vi "Get User Interface VI.vi"(8 "error in (no error)":errorcluster, 11 "DSF Buffer Converter Transfers UI in":refnum<class "Default Buffer Converter Transfers UI.lvclass">) -> (0 "error out":errorcluster, 2 "user interface vi":refnum<vi>, 3 "DSF Buffer Converter Transfers UI out":refnum<class "Default Buffer Converter Transfers UI.lvclass">)   [LabVIEW 2020, in "DSF Core.lvlib" / "Default Buffer Converter Transfers UI.lvclass"]
uses:
  Default Buffer Converter Transfers UI.lvclass
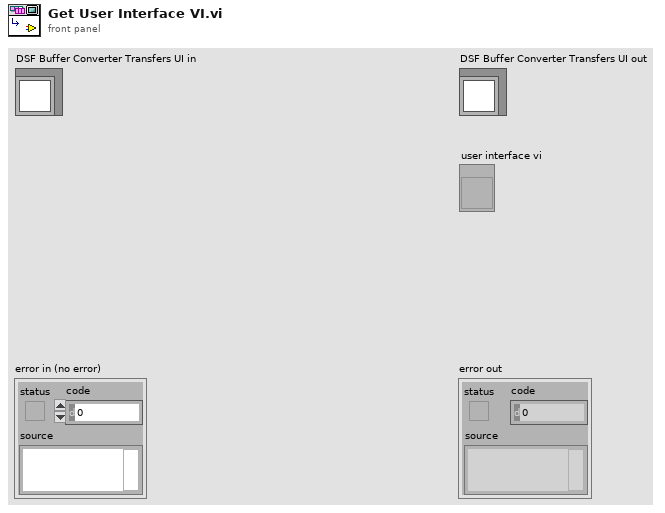
[diagram p1: front panel]
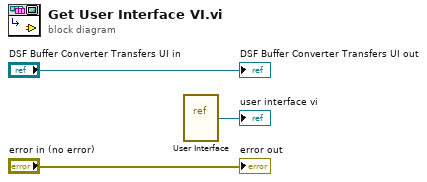
[diagram p0: block diagram]
diagram:
  n1 = vi-ref "User Interface.vi"() -> (→"user interface vi":refnum<vi>)
  "error out" <- "error in (no error)"
  "DSF Buffer Converter Transfers UI out" <- "DSF Buffer Converter Transfers UI in"
